vi "Percobaan 1.vi"() -> ()   [LabVIEW 2020]
uses:
  <vilib>/MakerHub/LINX/Public/Utilities/Open Serial.vi
  <vilib>/MakerHub/LINX/LMH-LINX.lvlib
  <vilib>/MakerHub/LINX/Public/Sensors/Distance/Ultrasonic/Ultrasonic.lvlib
panel:
  out "Jarak (cm)":dbl(slide) scale=0.0..100.0
  in  "stop":bool
  in  "Serial Port":refnum<visa-resource-name>
  # "Pengukuran Jarak-Ultrasonic sensor"
  # "EK-2B\n1. Aldisyah Putra Mahardika   \t\t\n(EK-2B/3.32.21.1.02) \n2. Aurelia Alika Putri Widiyanta  \t\n(EK-2B/3.32.21.1.04) \n3. Fahmi Fathur Rohman     \t\t\n(EK-2B/3.32.21.1.08)"
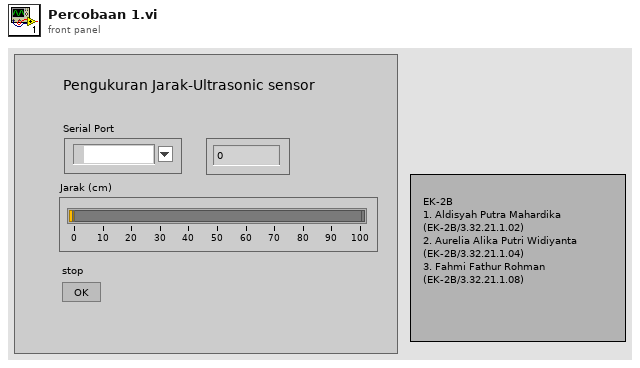
[diagram p1: front panel]
types:
  T1 = typedef "LMH-LINX.lvlib/LINX Ref.ctl" = cluster{"IO":T2, "Interface":T3, "LINX Device Config":T4}
  T2 = typedef "LMH-LINX.lvlib/Platform.ctl" = enum16{"Remote", "Local"}
  T3 = typedef "LMH-LINX.lvlib/Interface.ctl" = enum16{"Serial", "TCP"}
  T4 = typedef "LMH-LINX.lvlib/Device.lvlib/LINX Device Config.ctl" = cluster{"Interface":T3, "COM Port":refnum<visa-resource-name>, "TCP Configuration":T5, "Device Family":u8, "Device ID":u8, "Device Name":string, "TCP Ref":refnum<k5>, "Channels":T6}
  T5 = typedef "LMH-LINX.lvlib/Device.lvlib/TCP Config.ctl" = cluster{"IP Address":string, "Port":u16}
  T6 = typedef "LMH-LINX.lvlib/Channels.ctl" = cluster{"DI":u8[], "DO":u8[], "AI":u8[], "AO":u8[], "PWM":u8[], "QE":u8[], "UART":u8[], "I2C 2":u8[], "SPI":u8[], "CAN":u8[], "Servo":u8[], "AI Ref (V)":dbl, "AI Resolution (Bits)":u8, "AO Ref (V)":dbl, "AO Resolution (Bits)":u8}
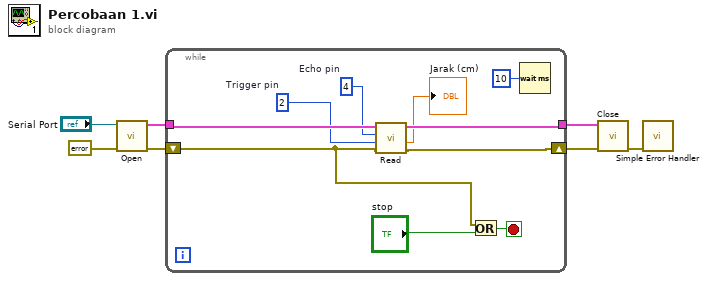
[diagram p0: block diagram]
diagram:
  n1 = call-poly <vilib>:"Open.vi"("Error In"=errorcluster {"status"=FALSE, "code"=0, "source"=""}, "Serial Port"="Serial Port") -> ("Error Out"=w7:errorcluster, "LINX Resource"=w1:T1)  [unwired: 7 in, 1 out]
  n2 = while {
    tunnel: w1 -> [w11]
    tunnel: [w14] -> w6
    shift-right: [w13] -> w5
    shift-left: w7 -> [w12]
    stop <- w17 stop-if-true
    w9 = u8 4  # Echo pin
    w10 = u8 2  # Trigger pin
    n3 = call <vilib>:"Read.vi"("Error In"=w12, "DO Channel"=w10, "DI Channel"=w9, "LINX Resource"=w11) -> ("Error Out"=w13:errorcluster, "Centimeters"=→"Jarak (cm)":dbl, "LINX Resource"=w14:T1)  [unwired: 4 in, 1 out]
    n4 = Or(x=w12, y="stop") -> (x .or. y?=w17:bool)
    n5 = Wait (ms)(milliseconds to wait=u32 10) -> ()  [unwired: 1 out]
  }
  n6 = call <vilib>:"Close.vi"("Error In"=w5, "LINX Resource"=w6) -> ("Error Out"=w3:errorcluster)  [unwired: 9 in]
  n7 = call <vilib>:"Simple Error Handler.vi"("error in (no error)"=w3) -> ()  [unwired: 4 in, 5 out]
